vi "newTestStandGlobalVariable.vi"(0 "Engine Reference":refnum<k7>, 5 "Sequence File Ref":refnum<k7>, 7 "Variable Type":i32(ring)=1 items=["PropValType_Container", "PropValType_String", "PropValType_Boolean", "PropValType_Number", "PropValType_NamedType", "PropValType_Reference", "PropValType_Array"], 9 "Variable Name":string="Locals.Logs", 11 "error in":errorcluster, 12 "Array?":bool) -> (4 "Engine Reference(out)":refnum<k7>, 6 "Sequence File Ref(out)":refnum<k7>, 15 "error out":errorcluster)   [LabVIEW 2009]
panel:
  in  "Empty array?":bool
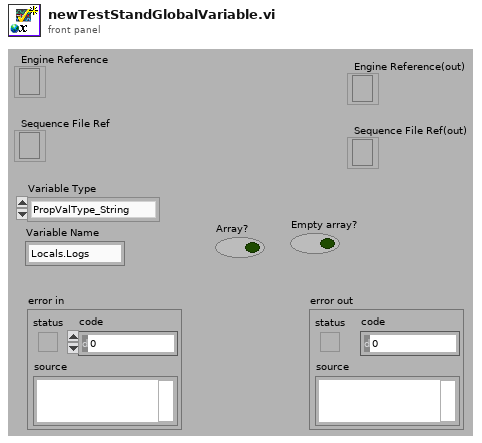
[diagram p1: front panel]
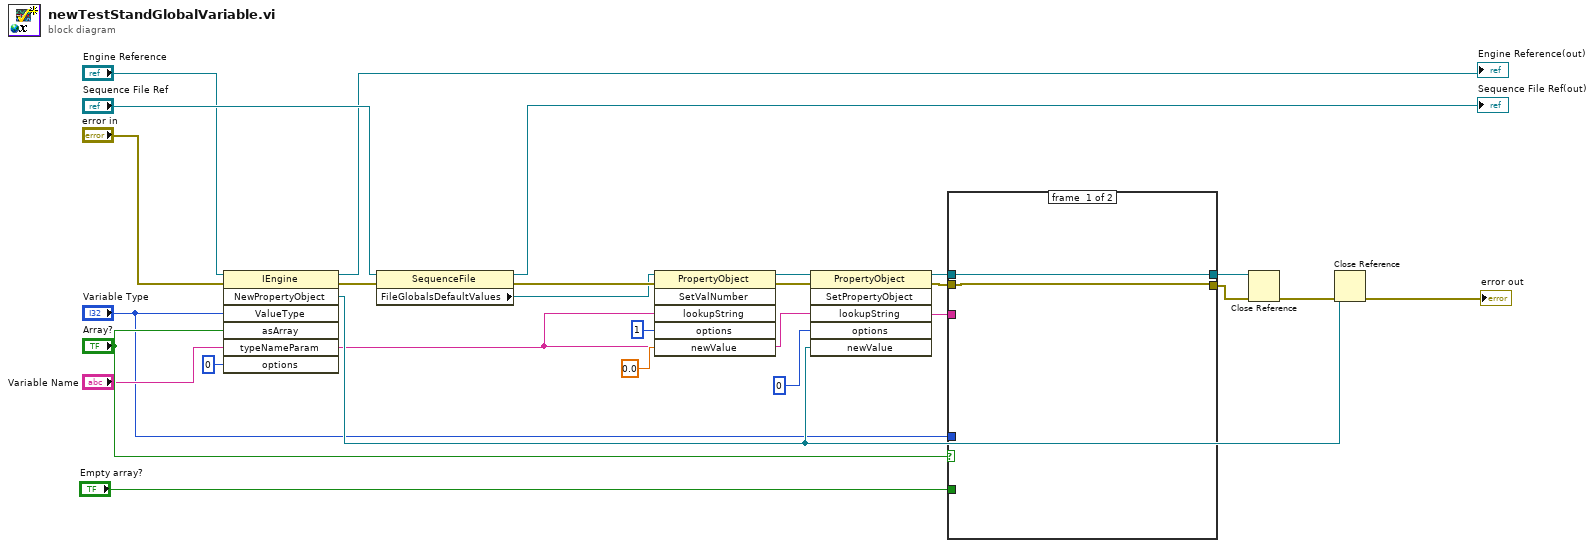
[diagram p0: block diagram]
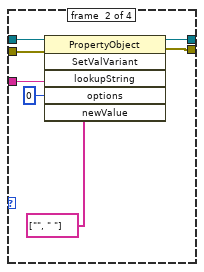
[diagram p3: hidden frame]
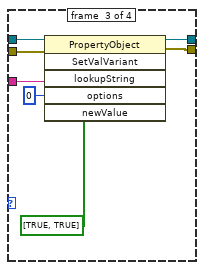
[diagram p4: hidden frame]
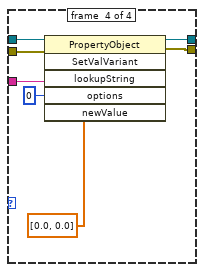
[diagram p5: hidden frame]
diagram:
  n1 = invoke class="IEngine" method="NewPropertyObject"(reference="Engine Reference", error in="error in", "ValueType"="Variable Type", "asArray"="Array?", "typeNameParam"="Variable Name", "options"=0) -> (reference out=→"Engine Reference(out)":refnum<k7>, error out=w13:errorcluster, "NewPropertyObject"=w12:refnum<k7>)  [unwired: 1 in, 4 out]
  n2 = property class="SequenceFile"(reference="Sequence File Ref", error in=w13) -> (reference out=→"Sequence File Ref(out)":refnum<k7>, error out=w3:errorcluster, "FileGlobalsDefaultValues"=w2:refnum<k7>)
  n3 = invoke class="PropertyObject" method="SetValNumber"(reference=w2, error in=w3, "lookupString"="Variable Name", "options"=1, "newValue"=0.0) -> (reference out=w18:refnum<k7>, error out=w16:errorcluster)  [unwired: 1 in, 4 out]
  n4 = invoke class="PropertyObject" method="SetPropertyObject"(reference=w18, error in=w16, "lookupString"="Variable Name", "options"=0, "newValue"=w12) -> (reference out=w10:refnum<k7>, error out=w7:errorcluster)  [unwired: 1 in, 4 out]
  n5 = case shown="True" "Array?" {
    tunnel: w10 -> [w27 w34]
    tunnel: [w27 w33] -> w9
    tunnel: "Empty array?" -> [_ w30]
    tunnel: [w26 w31] -> w6
    tunnel: w7 -> [w26 w32]
    tunnel: "Variable Name" -> [_ w29]
    tunnel: "Variable Type" -> [_ w28]
    frame #0 {
    }
    frame #1 {
      n6 = case shown="False" w30 {
        tunnel: w34 -> [w40 w65]
        tunnel: [w36 w65] -> w33
        tunnel: w32 -> [w39 w64]
        tunnel: [w35 w64] -> w31
        tunnel: w29 -> [w38 _]
        tunnel: w28 -> [w37 _]
        frame #0 {
          n7 = case shown="2" w37 {
            tunnel: w40 -> [w42 w49 w56 w63]
            tunnel: w39 -> [w41 w48 w55 w62]
            tunnel: w38 -> [_ w47 w54 w61]
            tunnel: [w42 w46 w53 w60] -> w36
            tunnel: [w41 w45 w52 w59] -> w35
            frame #0 {
            }
            frame #1 {
              n8 = invoke class="PropertyObject" method="SetValVariant"(reference=w49, error in=w48, "lookupString"=w47, "options"=0, "newValue"=string[] ["", " "]) -> (reference out=w46:refnum<k7>, error out=w45:errorcluster)  [unwired: 1 in, 4 out]
            }
            frame #2 {
              n9 = invoke class="PropertyObject" method="SetValVariant"(reference=w56, error in=w55, "lookupString"=w54, "options"=0, "newValue"=bool[] [TRUE, TRUE]) -> (reference out=w53:refnum<k7>, error out=w52:errorcluster)  [unwired: 1 in, 4 out]
            }
            frame #3 {
              n10 = invoke class="PropertyObject" method="SetValVariant"(reference=w63, error in=w62, "lookupString"=w61, "options"=0, "newValue"=dbl[] [0.0, 0.0]) -> (reference out=w60:refnum<k7>, error out=w59:errorcluster)  [unwired: 1 in, 4 out]
            }
          }
        }
        frame #1 {
        }
      }
    }
  }
  n11 = Close Reference(reference=w9, error in (no error)=w6) -> (error out=w1:errorcluster)
  n12 = Close Reference(reference=w12, error in (no error)=w1) -> (error out=→"error out":errorcluster)
